vi "Graf pre User dfefined FINAL.vi"(1 "Array":dbl[](array[numeric]), 2 "Array 2":i16[](array[numeric])) -> (0 "Boolean":bool)   [LabVIEW 2018]
panel:
  out "po prevode 3":i16[](graph)
  in  "Zrusit":bool
  in  "OK Button":bool
  out "po prevode 2":dbl[](graph)
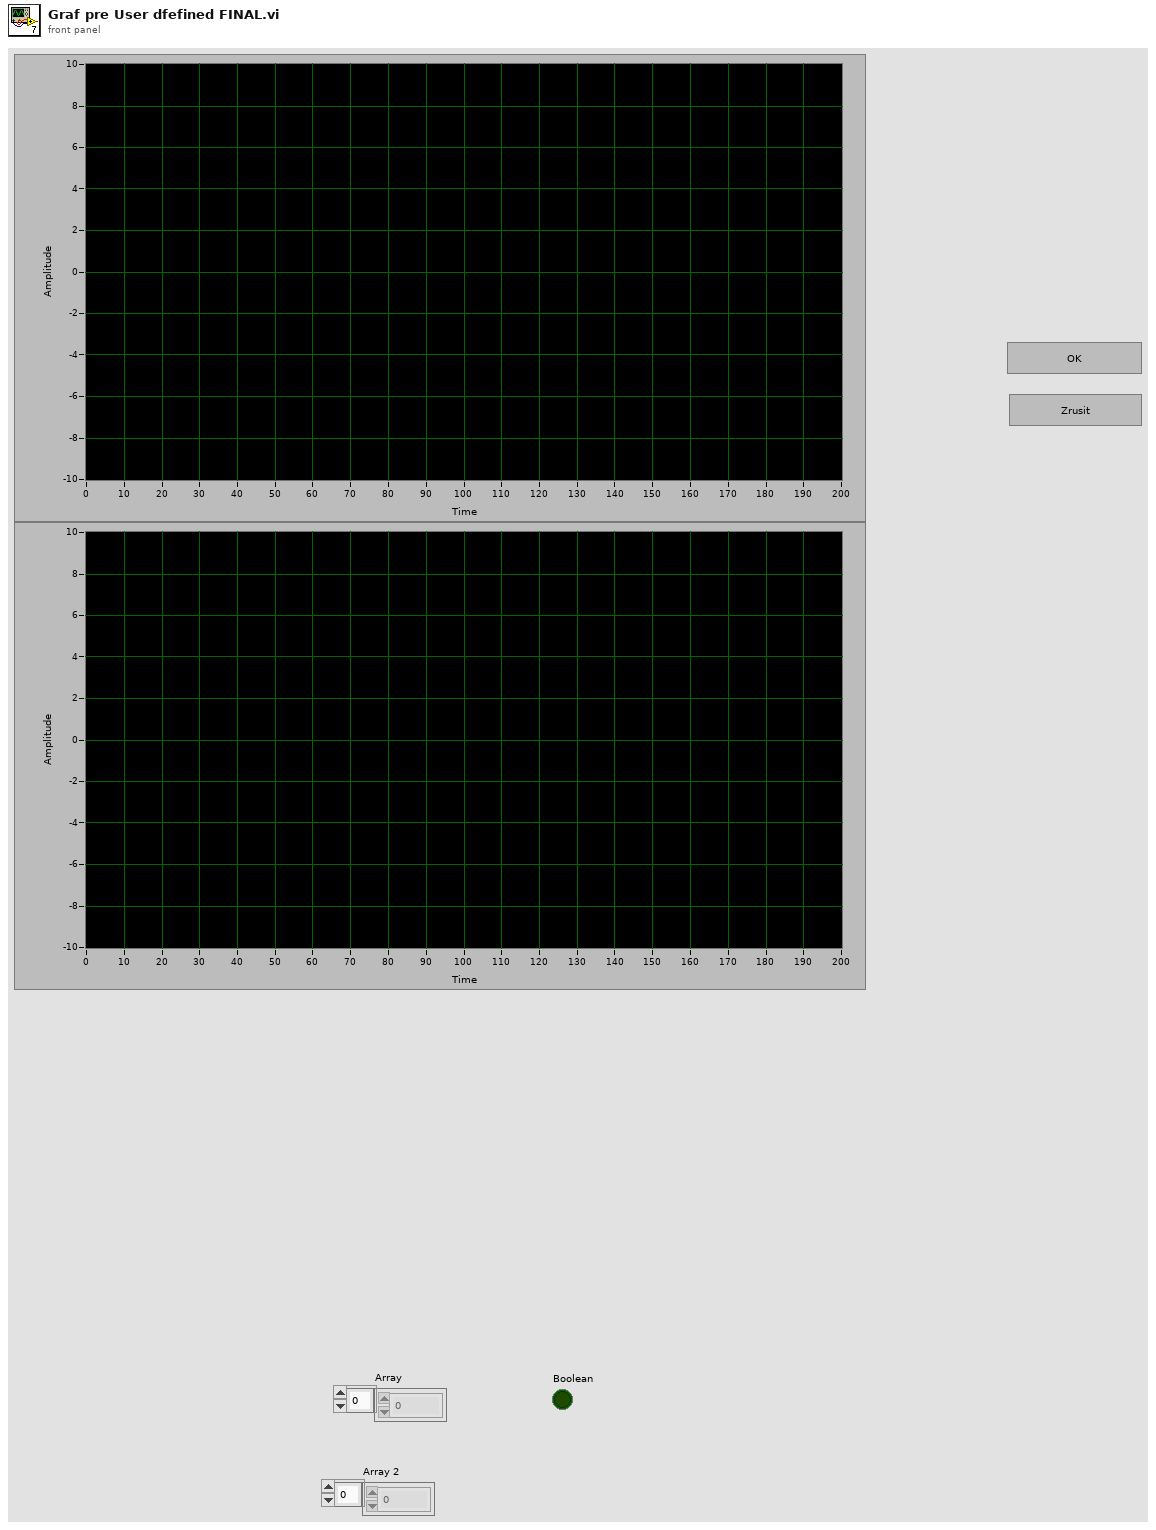
[diagram p1: front panel]
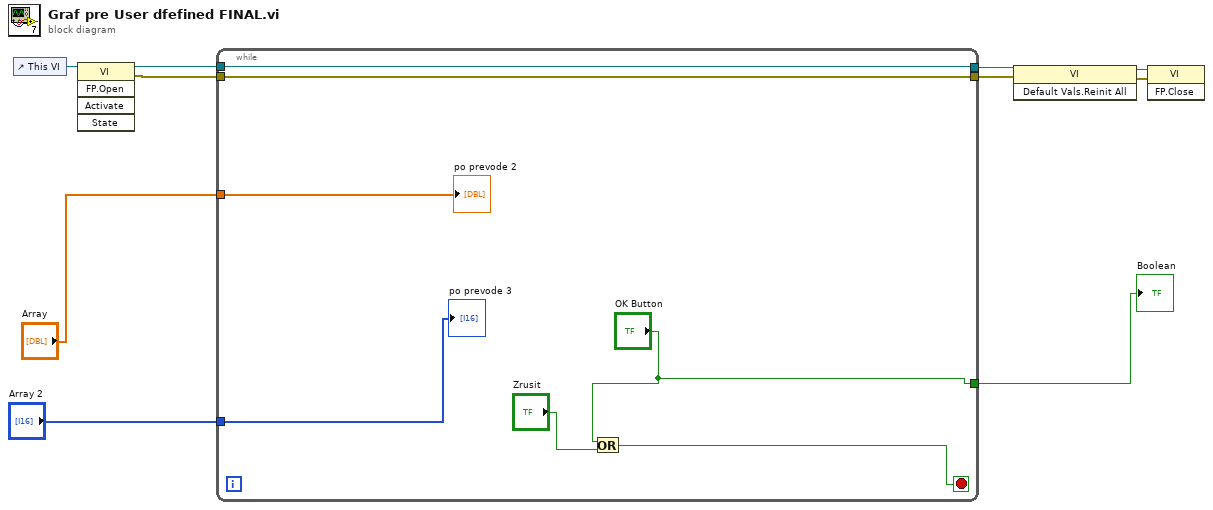
[diagram p0: block diagram]
diagram:
  n1 = control-ref of="This VI"() -> (w10:refnum<vi>)
  n2 = invoke class="VI" method="FP.Open"(reference=w10) -> (reference out=w9:refnum<vi>, error out=w8:errorcluster)  [unwired: 4 in, 3 out]
  n3 = while {
    tunnel: [w17] -> w5
    tunnel: w9 -> [w17]
    tunnel: [w16] -> w4
    tunnel: w8 -> [w16]
    tunnel: "Array" -> [w15]
    tunnel: ["OK Button"] -> w2
    tunnel: "Array 2" -> [w11]
    stop <- w13 stop-if-true
    n4 = Or(x="OK Button", y="Zrusit") -> (x .or. y?=w13:bool)
    "po prevode 2" <- w15
    "po prevode 3" <- w11
  }
  "Boolean" <- w2
  n5 = invoke class="VI" method="Default Vals.Reinit All"(reference=w5, error in=w4) -> (reference out=w7:refnum<vi>, error out=w6:errorcluster)  [unwired: 1 in, 1 out]
  n6 = invoke class="VI" method="FP.Close"(reference=w7, error in=w6) -> ()  [unwired: 1 in, 3 out]
